vi "Select email recipient.vi"(8 "error in (no error)":errorcluster, 10 "Recipient file":path, 11 "email recipients":string[](array[string])) -> (0 "error out":errorcluster, 3 "Email recipient":string)   [LabVIEW 2013]
panel:
  in  "Add to list":bool
  in  "Email recipients":i32(listbox)
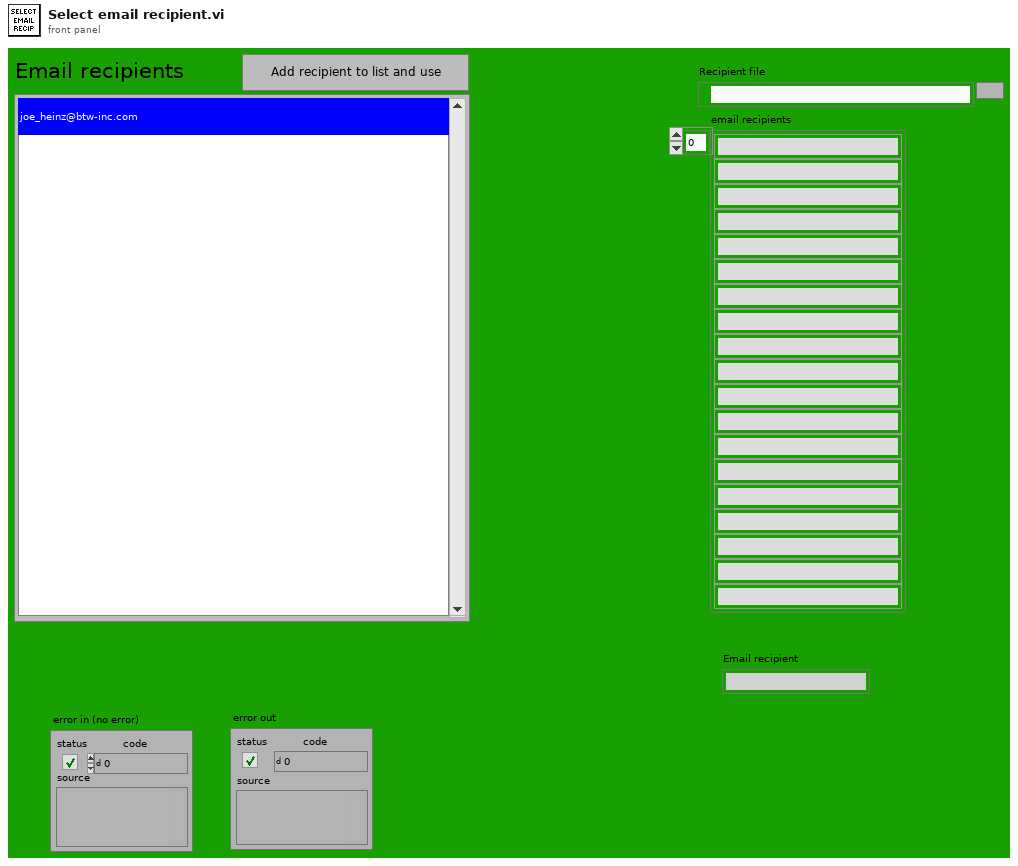
[diagram p1: front panel]
types:
  T1 = enum16{"open", "replace", "create", "open or create", "replace or create", "replace or create with confirmation"}
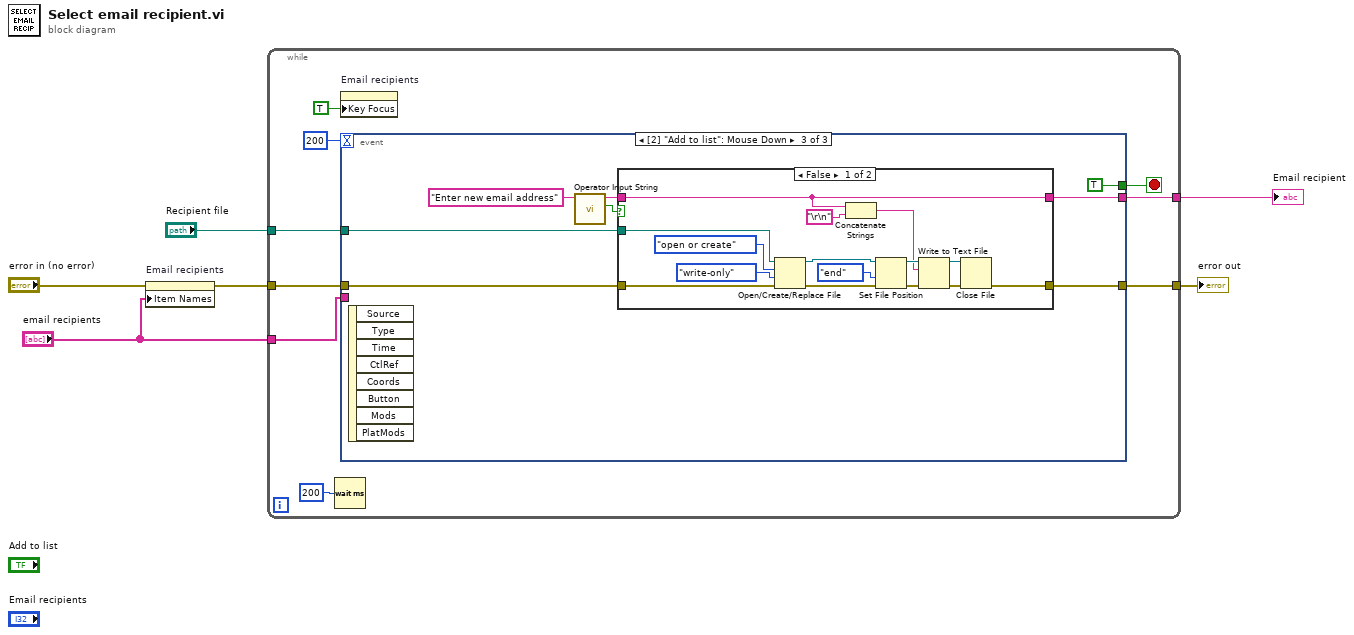
[diagram p0: block diagram]
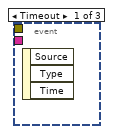
[diagram p2: hidden frame]
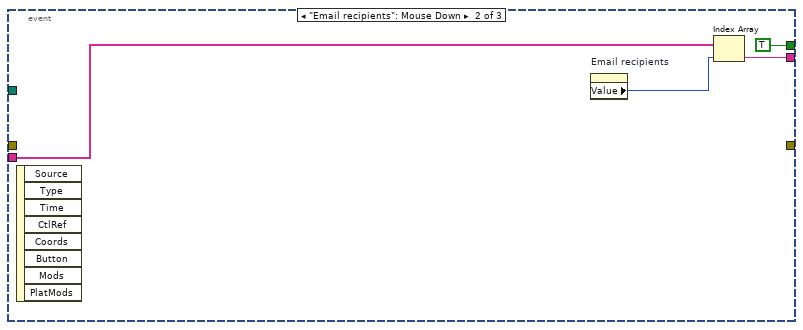
[diagram p3: hidden frame]
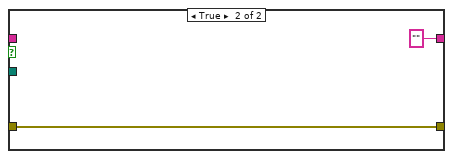
[diagram p4: hidden frame]
diagram:
  n1 = property on="Email recipients" class="LstBox (strict)"(error in="error in (no error)", "Item Names"="email recipients") -> (error out=w2:errorcluster)  [unwired: 1 in, 1 out]
  n2 = while {
    tunnel: "email recipients" -> [w10]
    tunnel: [w11] -> w5
    tunnel: [w7] -> w4
    tunnel: w2 -> [w8]
    tunnel: "Recipient file" -> [w9]
    stop <- w12 stop-if-true
    n3 = Wait (ms)(milliseconds to wait=u32 200) -> ()  [unwired: 1 out]
    n4 = property on="Email recipients" class="LstBox (strict)"("Key Focus"=TRUE) -> ()  [unwired: 2 in, 2 out]
    n5 = event shown="[2] \"Add to list\": Mouse Down" {
      selector: _ -> [_ _ _]
      dyn-events: _ -> [_ _ _]
      timeout: 200 -> [_ _ _]
      tunnel: [_ TRUE ("Key Focus") TRUE ("Key Focus")] -> w12
      tunnel: w10 -> [_ w17 _]
      tunnel: [_ w16 w26] -> w11
      tunnel: w9 -> [_ _ w25]
      tunnel: w8 -> [_ _ w21]
      tunnel: [_ _ w20] -> w7
      event Timeout {
        n6 = event-data() -> ()  [unwired: 1 in, 3 out]
      }
      event "Email recipients": Mouse Down {
        n7 = event-data() -> ()  [unwired: 1 in, 8 out]
        n8 = property on="Email recipients" class="LstBox (strict)"() -> ("Value"=w18:i32)  [unwired: 2 in, 2 out]
        n9 = Index Array(array=w17, index=w18) -> (element=w16:string)
      }
      event "Add to list": Mouse Down {
        n10 = event-data() -> ()  [unwired: 1 in, 8 out]
        n11 = call "Operator Input String.vi"("Message"="Enter new email address") -> ("Stop button hit"=w23:bool, "Response"=w22:string)  [unwired: 8 in, 1 out]
        n12 = case shown="False" w23 {
          tunnel: w22 -> [w30 _]
          tunnel: [w30 "" ("Response")] -> w26
          tunnel: w25 -> [w42 _]
          tunnel: w21 -> [w29 w43]
          tunnel: [w28 w43] -> w20
          frame False {
            n13 = Open/Create/Replace File(file path (use dialog)=w42, error in=w29, operation (0:open)=T1."open or create", access (0:read/write)=enum16{"read/write", "read-only", "write-only"}."write-only") -> (refnum out=w38:refnum<file>, error out=w39:errorcluster)  [unwired: 2 in, 1 out]
            n14 = Concatenate Strings(w30, "\r\n") -> (w33:string)
            n15 = Set File Position(refnum=w38, from (0:start)=enum16{"start", "end", "current"}."end", error in=w39) -> (refnum out=w34:refnum<file>, error out=w35:errorcluster)  [unwired: 1 in]
            n16 = Write to Text File(file (use dialog)=w34, text=w33, error in=w35) -> (refnum out=w31:refnum<file>, error out=w32:errorcluster)  [unwired: 1 in, 1 out]
            n17 = Close File(refnum=w31, error in=w32) -> (error out=w28:errorcluster)  [unwired: 1 out]
          }
          frame True {
          }
        }
      }
    }
  }
  "error out" <- w4
  "Email recipient" <- w5
